vi "PLC.WritePCData.vi"(8 "error in (no error)":errorcluster, 9 "Sets":T1, 10 "PCdata in":T2, 11 "Ref in":u64) -> (0 "error out":errorcluster, 2 "PCdata out":T2, 3 "Ref out":u64)   [LabVIEW 2016]
doc: "Write data block from PC to PLC\n\nWabco 2017 All right reserved\nAuthor: maciej.szupienko@wabco-auto.com"
uses:
  PLC.DataBlock.PCstatus.ctl
  PLC.DataBlock.PCstatus.General.ctl
  PLC.DataBlock.PCstatus.Station.ctl
  PLC.Data.Sets.ctl
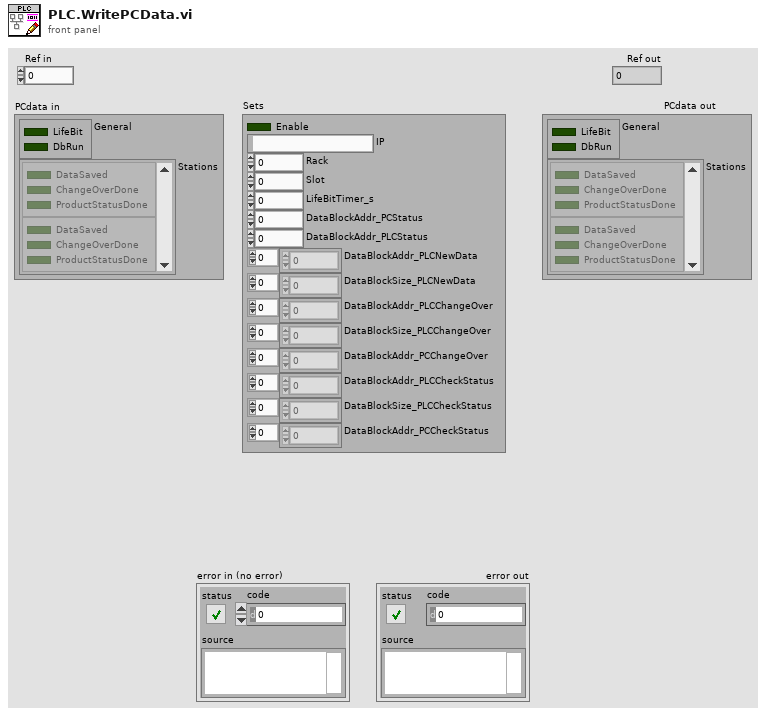
[diagram p1: front panel]
types:
  T1 = typedef "PLC.Data.Sets.ctl" = cluster{"Enable":bool, "IP":string, "Rack":i32, "Slot":i32, "LifeBitTimer_s":dbl, "DataBlockAddr_PCStatus":i32, "DataBlockAddr_PLCStatus":i32, "DataBlockAddr_PLCNewData":i32[], "DataBlockSize_PLCNewData":i32[], "DataBlockAddr_PLCChangeOver":i32[], "DataBlockSize_PLCChangeOver":i32[], "DataBlockAddr_PCChangeOver":i32[], "DataBlockAddr_PLCCheckStatus":i32[], "DataBlockSize_PLCCheckStatus":i32[], "DataBlockAddr_PCCheckStatus":i32[]}
  T2 = typedef "PLC.DataBlock.PCstatus.ctl" = cluster{"General":T3, "Stations":T4[]}
  T3 = typedef "PLC.DataBlock.PCstatus.General.ctl" = cluster{"LifeBit":bool, "DbRun":bool}
  T4 = typedef "PLC.DataBlock.PCstatus.Station.ctl" = cluster{"DataSaved":bool, "ChangeOverDone":bool, "ProductStatusDone":bool}
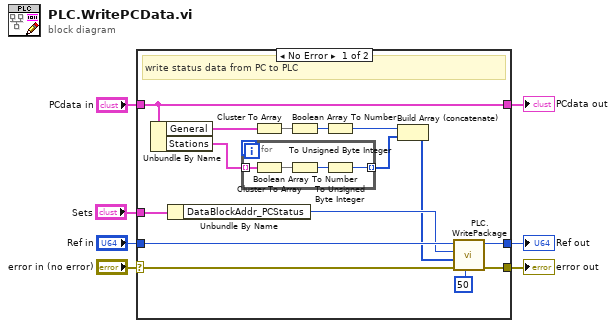
[diagram p0: block diagram]
diagram:
  n1 = case shown="No Error" "error in (no error)" {
    selector: "error in (no error)" -> [w13 w29]
    tunnel: "Ref in" -> [w14 w28]
    tunnel: [w11 w29] -> w6
    tunnel: "PCdata in" -> [w18 w27]
    tunnel: [w18 w27] -> w4
    tunnel: [w12 w28] -> w3
    tunnel: "Sets" -> [w22 _]
    frame No Error {
      # "write status data from PC to PLC"
      n2 = Unbundle By Name(w18) -> ("General"=w19:T3, "Stations"=w15:T4[])
      n3 = Unbundle By Name(w22) -> ("DataBlockAddr_PCStatus"=w9:i32)
      n4 = for {
        tunnel: w15 -> [w24] mode=indexing
        tunnel: [w23] -> w16 mode=indexing
        n5 = Cluster To Array(cluster=w24) -> (array=w25:bool[])
        n6 = Boolean Array To Number(Boolean array=w25) -> (number=w26:u32)
        n7 = To Unsigned Byte Integer(number=w26) -> (unsigned 8bit integer=w23:u8)
      }
      n8 = Cluster To Array(cluster=w19) -> (array=w21:bool[])
      n9 = Boolean Array To Number(Boolean array=w21) -> (number=w20:u32)
      n10 = To Unsigned Byte Integer(number=w20) -> (unsigned 8bit integer=w17:u8)
      n11 = Build Array (concatenate)(w17, w16) -> (w8:u8[])
      n12 = call "PLC.WritePackage.vi"("max package size  (0: full)"=50 ("max package size"), "error in (no error)"=w13, "data"=w8, "addr"=w9, "Ref in"=w14) -> ("error out"=w11:errorcluster, "Ref out"=w12:u64)  [unwired: 5 in]
    }
    frame Error {
    }
  }
  "PCdata out" <- w4
  "error out" <- w6
  "Ref out" <- w3
